vi "Read Offset.vi"(8 "error in":errorcluster, 10 "Offset Name":string, 11 "Config Folder":path) -> (0 "error out":errorcluster, 2 "Vec3d out":refnum<class "Vec3d Class.lvclass">)   [LabVIEW 2011]
uses:
  Vec3d Class/Vec3d Class.lvclass
  <vilib>/Utility/config.llb/Read Key (String).vi
  <vilib>/Utility/config.llb/NI_LVConfig.lvlib
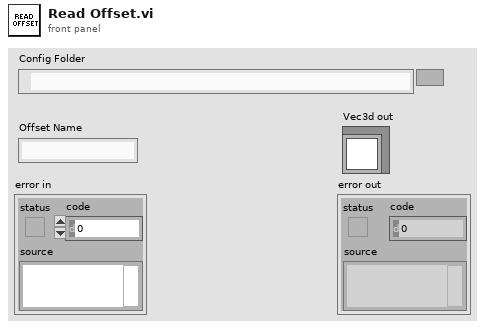
[diagram p1: front panel]
types:
  T1 = typedef "NI_LVConfig.lvlib/Config Data RefNum.ctl" = refnum<k1>
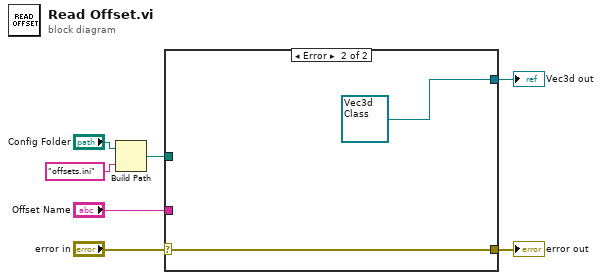
[diagram p0: block diagram]
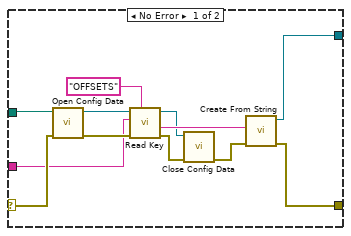
[diagram p2: hidden frame]
diagram:
  n1 = Build Path(base path="Config Folder", name or relative path="offsets.ini") -> (appended path=w3:path)
  n2 = case shown="Error" "error in" {
    selector: "error in" -> [w14 w21]
    tunnel: [w8 w21] -> w6
    tunnel: [w11 refnum<class "Vec3d Class.lvclass"> refnum ("Vec3d out")] -> w1
    tunnel: w3 -> [w19 _]
    tunnel: "Offset Name" -> [w13 _]
    frame No Error {
      n3 = call <vilib>:"Open Config Data.vi"("error in (no error)"=w14, "configuration file path"=w19) -> ("error out"=w16:errorcluster, "refnum"=w18:T1)  [unwired: 7 in, 1 out]
      n4 = call-poly <vilib>:"Read Key.vi"("section"="OFFSETS", "error in (no error)"=w16, "key"=w13, "refnum"=w18) -> ("error out"=w10:errorcluster, "value"=w17:string, "refnum out"=w12:T1)  [unwired: 4 in, 1 out]
      n5 = call <vilib>:"Close Config Data.vi"("error in (no error)"=w10, "refnum"=w12) -> ("error out"=w9:errorcluster)  [unwired: 8 in, 1 out]
      n6 = call "Create From String.vi"("error in"=w9, "Input String"=w17) -> ("error out"=w8:errorcluster, "Vec3d out"=w11:refnum<class "Vec3d Class.lvclass">)  [unwired: 8 in]
    }
    frame Error {
    }
  }
  "error out" <- w6
  "Vec3d out" <- w1
